vi "Read Number of Measurements.vi"(11 "MCCW ACLR in":refnum<class "MCCW ACLR.lvclass">) -> (2 "Number of Measurements":T1, 3 "MCCW ACLR out":refnum<class "MCCW ACLR.lvclass">)   [LabVIEW 2020, in "MCCW ACLR.lvclass"]
uses:
  MCCW ACLR.lvclass
  MCCW ACLR.lvclass/MCCW ACLR.ctl
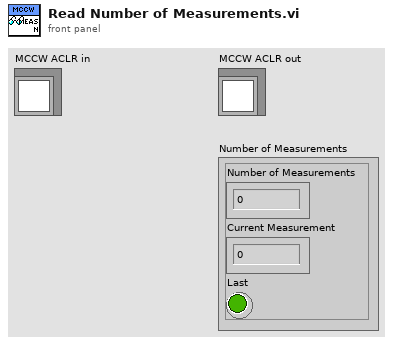
[diagram p1: front panel]
types:
  T1 = cluster{"Number of Measurements":u32, "Current Measurement":u32, "Last":bool}
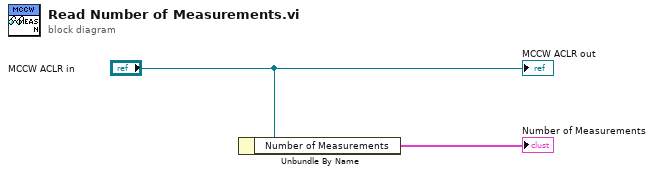
[diagram p0: block diagram]
diagram:
  n1 = Unbundle By Name("MCCW ACLR in") -> ("Number of Measurements"=→"Number of Measurements":T1)
  "MCCW ACLR out" <- "MCCW ACLR in"
